vi "InitNumericValuesFromRegistry(SubVI).vi"(4 "error in (no error)":errorcluster, 5 "Numeric References":refnum<vi>[](array[refnum]), 6 "subkey":string, 7 "root key (HKEY_LOCAL_MACHINE)":T1) -> (0 "error out":errorcluster, 1 "Numeric Values":dbl[](array[numeric]), 2 "Key Values":string[](array[string]), 3 "Control Labels":string[](array[string]))   [LabVIEW 2010]
uses:
  <vilib>/registry/registry.llb/Registry RtKey.ctl
  <vilib>/registry/registry.llb/Registry SAM.ctl
  <vilib>/registry/registry.llb/Read Registry Value Simple STR.vi
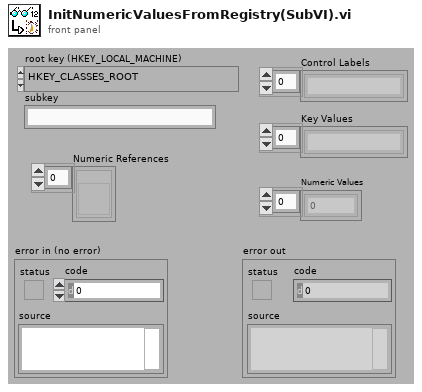
[diagram p1: front panel]
types:
  T1 = typedef "Registry RtKey.ctl" = enum32{"HKEY_CLASSES_ROOT", "HKEY_CURRENT_USER", "HKEY_LOCAL_MACHINE", "HKEY_USERS", "HKEY_PERFORMANCE_DATA", "HKEY_CURRENT_CONFIG", "HKEY_DYN_DATA"}
  T2 = typedef "Registry SAM.ctl" = enum32{"KEY_QUERY_VALUE", "KEY_SET_VALUE", "KEY_CREATE_SUB_KEY", "KEY_ENUMERATE_SUB_KEYS", "KEY_NOTIFY", "KEY_CREATE_LINK", "KEY_READ", "KEY_WRITE", "KEY_ALL_ACCESS", "KEY_READ | KEY_WRITE"}
  T3 = typedef "Registry refnum.ctl" = refnum<k1>
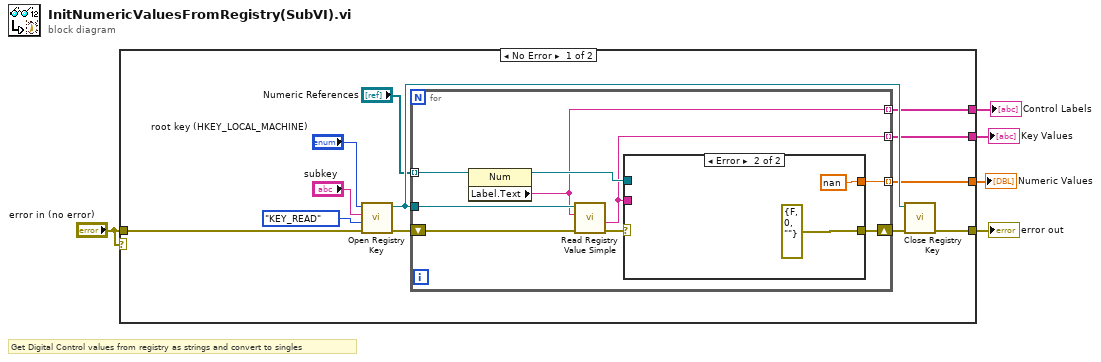
[diagram p0: block diagram]
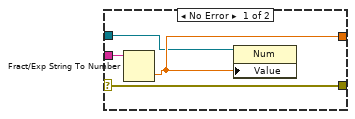
[diagram p2: hidden frame]
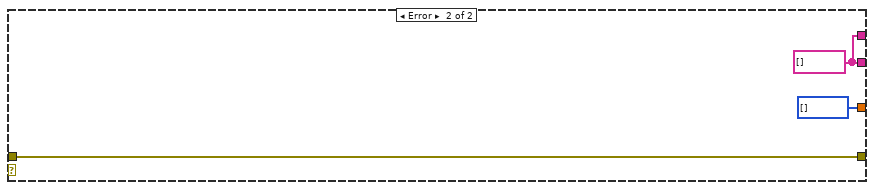
[diagram p3: hidden frame]
diagram:
  # "Get Digital Control values from registry as strings and convert to singles"
  n1 = case shown="No Error" "error in (no error)" {
    tunnel: "error in (no error)" -> [w10 w35]
    tunnel: [w9 w35] -> w4
    tunnel: [w8 w34] -> w3
    tunnel: [w7 w34] -> w2
    tunnel: [w6 i32[] []] -> w1
    frame No Error {
      n2 = call <vilib>:"Open Registry Key.vi"("error in (no error)"=w10, "security access mask (KEY_READ | KEY_WRITE)"=Registry_SAM."KEY_READ", "subkey"="subkey", "root key (HKEY_LOCAL_MACHINE)"="root key (HKEY_LOCAL_MACHINE)") -> ("error out"=w15:errorcluster, "refnum out"=w16:T3)  [unwired: 6 out]
      n3 = for {
        tunnel: "Numeric References" -> [w25] mode=indexing
        shift-right: [w21] -> w17
        shift-left: w15 -> [w24]
        tunnel: w16 -> [w23]
        tunnel: [w20] -> w8 mode=indexing
        tunnel: [w19] -> w7 mode=indexing
        tunnel: [w18] -> w6 mode=indexing
        n4 = property class="Num"(reference=w25) -> (reference out=w26:refnum<vi>, "Label.Text"=w20:string)  [unwired: 1 in, 1 out]
        n5 = call-poly <vilib>:"Read Registry Value Simple.vi"("error in (no error)"=w24, "value"=w20, "refnum"=w23) -> ("error out"=w22:errorcluster, "String/Binary data"=w19:string)  [unwired: 1 in, 4 out]
        n6 = case shown="Error" w22 {
          selector: w22 -> [w29 _]
          tunnel: w26 -> [w27 _]
          tunnel: w19 -> [w30 _]
          tunnel: [w29 errorcluster {"status"=FALSE, "code"=0, "source"=""} ("error IO")] -> w21
          tunnel: [w28 nan] -> w18
          frame No Error {
            n7 = Fract/Exp String To Number(string=w30) -> (number=w28:dbl)  [unwired: 4 out]
            n8 = property class="Num"(reference=w27, "Value"=w28) -> ()  [unwired: 1 in, 2 out]
          }
          frame Error {
          }
        }
      }
      n9 = call <vilib>:"Close Registry Key.vi"("error in (no error)"=w17, "refnum"=w16) -> ("error out"=w9:errorcluster)  [unwired: 5 out]
    }
    frame Error {
      w34 = string[] []
    }
  }
  "error out" <- w4
  "Control Labels" <- w3
  "Key Values" <- w2
  "Numeric Values" <- w1
